vi "Write Gas Ref.vi"(8 "error in":errorcluster, 10 "Gas Ref":refnum<data-value>, 11 "Particle Properties in":refnum<class "Particle Properties.lvclass">) -> (0 "error out":errorcluster, 3 "Particle Properties out":refnum<class "Particle Properties.lvclass">)   [LabVIEW 2015, in "Particle Properties.lvclass"]
uses:
  Particle Properties.lvclass
  Atmospheric/Gas Properties/Gas Properties.lvclass
  Particle Properties.lvclass/Particle Properties.ctl
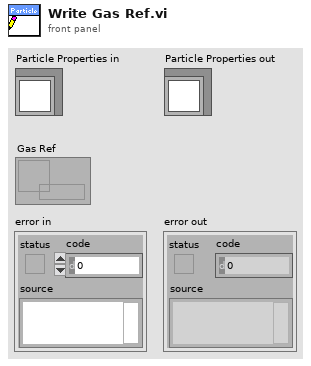
[diagram p1: front panel]
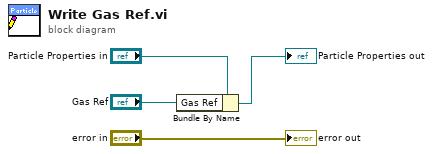
[diagram p0: block diagram]
diagram:
  n1 = Bundle By Name(cluster="Particle Properties in", "Gas Ref"="Gas Ref") -> (→"Particle Properties out":refnum<class "Particle Properties.lvclass">)
  "error out" <- "error in"
